vi "Map Column Indices.vi"(8 "error in (no error)":errorcluster, 10 "Index":i32, 11 "TestStand Result Handler in":refnum<class "TestStand Result Handler.lvclass">) -> (0 "error out":errorcluster, 2 "Mapped Index":i32, 3 "TestStand Result Handler out":refnum<class "TestStand Result Handler.lvclass">)   [LabVIEW 2020, in "Astemes_CSVReportPlugin.lvlib" / "TestStand Result Handler.lvclass"]
doc: "This VI is called when adding result data to a new row to map the collumn indices. \n\nThis is provided as a hook to modify the report by creating a sub-class of the Result Handler. If additional columns are inserted into the report, this VI needs to be implemented to map the default columns to the new indices."
uses:
  TestStand Result Handler.lvclass
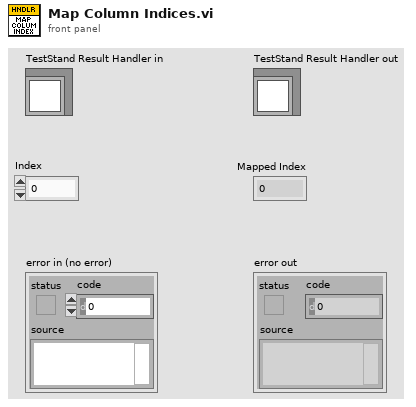
[diagram p1: front panel]
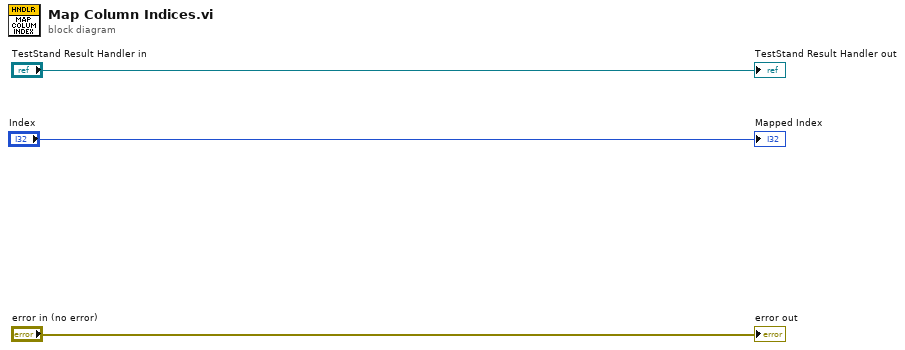
[diagram p0: block diagram]
diagram:
  "error out" <- "error in (no error)"
  "TestStand Result Handler out" <- "TestStand Result Handler in"
  "Mapped Index" <- "Index"
